vi "Autonomous Independent.vi"   [LabVIEW 2020]
doc: "This VI is called when autonomous begins, and will automatically be terminated when autonomous ends. You can carry out timed or sensor driven robot movement independently without needing to return to the caller."
uses:
  <vilib>/Rock Robotics/WPI/Solenoid/WPI_SolenoidValue.ctl
  <vilib>/Rock Robotics/Network Tables/NT Read String.vi
  <vilib>/Rock Robotics/Network Tables/NT Write String.vi
  Robot Global Data.vi
  <vilib>/Rock Robotics/WPI/Solenoid/WPI_SolenoidSetEnum.vi
  <vilib>/Rock Robotics/Network Tables/NT Write Numeric Array.vi
panel:
  # "Be sure to right-click and choose Data Operations>>Make Current Value default if you want to save the array values with the VI"
types:
  T1 = typedef "WPI_JoystickDevRef.ctl" = cluster{"Device":T2}
  T2 = typedef "WPI_JoystickDeviceEnum.ctl" = enum16{"USB 0", "USB 1", "USB 2", "USB 3", "USB 4", "USB 5"}
  T3 = enum16{"No-op", "Auto_Balance", "Arm_Setpoint", "Gripper", "Turn_IMU", "Drive_Distance", "Drive_to_Roll", "Stow_Intake", "Drive_to_GO", "Drive_to_Grid"}
  T4 = enum16{"Manual", "High Cone", "High Cube", "Mid Cone", "Mid Cube", "Intake", "Cube Handoff", "Cone Handoff", "Stow"}
  T5 = typedef "WPI_SolenoidValue.ctl" = enum16{"Off", "On", "Forward", "Reverse"}
  T6 = typedef "WPI_SolenoidDevRef.ctl" = cluster{"DevStatus":errorcluster, "Pneumatics Control Module":u8, "Forward Solenoid Channel":T7, "Reverse Solenoid Channel":T7}
  T7 = typedef "WPI_SolenoidChannel.ctl" = enum8{"Solenoid 0", "Solenoid 1", "Solenoid 2", "Solenoid 3", "Solenoid 4", "Solenoid 5", "Solenoid 6", "Solenoid 7", "Solenoid 8", "Solenoid 9", "Solenoid 10", "Solenoid 11", "Solenoid 12", "Solenoid 13", "Solenoid 14", "Solenoid 15", "Invalid"}
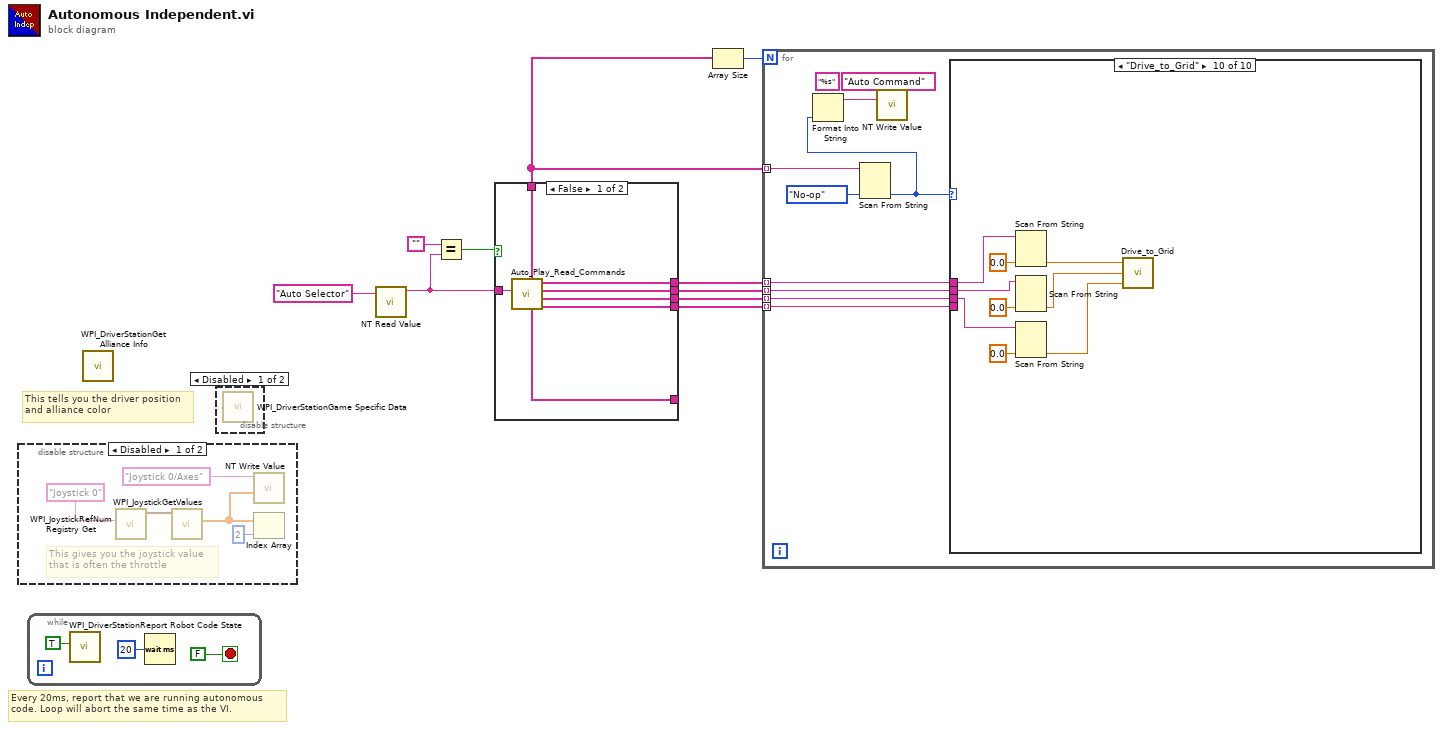
[diagram p0: block diagram]
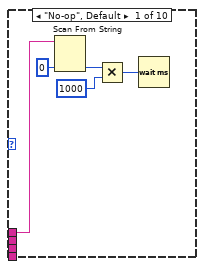
[diagram p2: hidden frame]
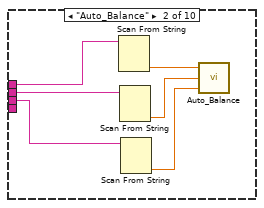
[diagram p3: hidden frame]
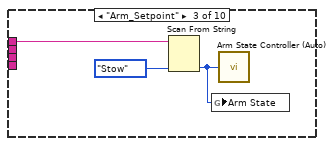
[diagram p4: hidden frame]
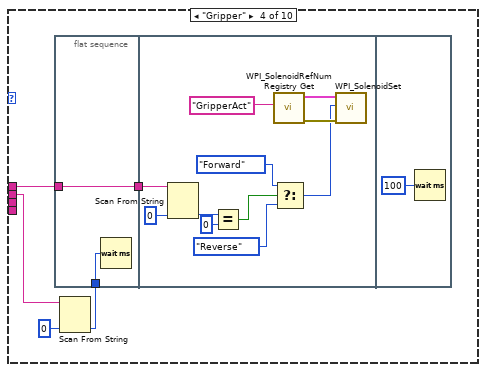
[diagram p5: hidden frame]
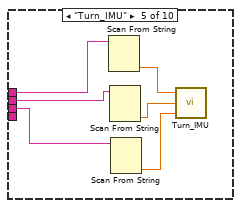
[diagram p6: hidden frame]
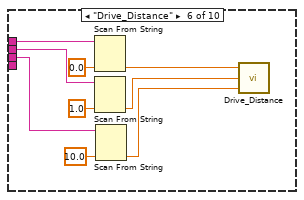
[diagram p7: hidden frame]
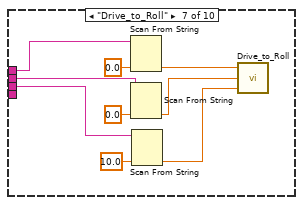
[diagram p8: hidden frame]
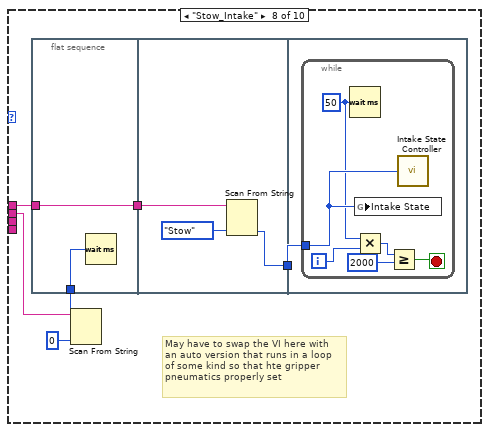
[diagram p9: hidden frame]
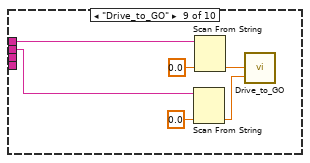
[diagram p10: hidden frame]
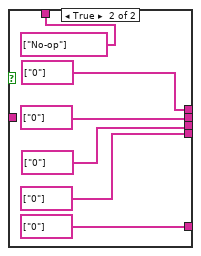
[diagram p11: hidden frame]
diagram:
  # "Every 20ms, report that we are running autonomous\ncode. Loop will abort the same time as the VI."
  # "This tells you the driver position\nand alliance color"
  n1 = disable-structure shown="Disabled" {
    frame Disabled {
      # "This gives you the joystick value\nthat is often the throttle"
      n2 = call <vilib>:"WPI_JoystickRefNum Registry Get.vi"("refnum name"="Joystick 0") -> ("JoystickDevRef"=w14:T1)  [unwired: 1 in, 9 out]
      n3 = call <vilib>:"WPI_JoystickGetValues.vi"("JoystickDevRef"=w14) -> ("Axes"=w12:dbl[])  [unwired: 6 in, 4 out]
      n4 = call-poly <vilib>:"NT Write Value.vi"("value"=w12, "name"="Joystick 0/Axes" ("Name")) -> ()  [unwired: 9 in, 1 out]
      n5 = Index Array(array=w12, index=2) -> ()  [unwired: 1 out]
    }
    frame Enabled {
    }
  }
  n6 = while {
    stop <- FALSE stop-if-true
    n7 = call <vilib>:"WPI_DriverStationReport Robot Code State.vi"("Autonomous"=TRUE) -> ()  [unwired: 10 in, 1 out]
    n8 = Wait (ms)(milliseconds to wait=u32 20) -> ()  [unwired: 1 out]
  }
  n9 = call <vilib>:"WPI_DriverStationGet Alliance Info.vi"() -> ()  [unwired: 12 out]
  n10 = disable-structure shown="Disabled" {
    frame Disabled {
      n11 = call <vilib>:"WPI_DriverStationGame Specific Data.vi"() -> ()  [unwired: 11 in, 1 out]
    }
    frame Enabled {
    }
  }
  n12 = call-poly <vilib>:"NT Read Value.vi"("name"="Auto Selector" ("Name")) -> ("value"=w7:string)  [unwired: 8 in, 2 out]
  n13 = Equal?(x="", y=w7) -> (x = y?=w8:bool)
  n14 = case shown="False" w8 {
    tunnel: w7 -> [w25 _]
    tunnel: [w24 string[] ["No-op"] ("Command Names")] -> w1
    tunnel: [w23 string[] ["0"] ("Parameter 1")] -> w5
    tunnel: [w22 string[] ["0"] ("Parameter 2")] -> w4
    tunnel: [w21 string[] ["0"] ("Parameter 3")] -> w3
    tunnel: [w20 string[] ["0"] ("Parameter 4")] -> w2
    tunnel: [w19 string[] ["0"] ("Concurrent?")] -> _
    frame False {
      n15 = call "Auto_Play_Read_Commands.vi"("Play Name"=w25) -> ("Parameter 4"=w20:string[], "Parameter 3"=w21:string[], "Parameter 2"=w22:string[], "Parameter 1"=w23:string[], "Concurrent?"=w19:string[], "Command Names"=w24:string[])  [unwired: 5 in]
    }
    frame True {
    }
  }
  n16 = Array Size(array=w1) -> (size(s)=w6:i32)
  n17 = for {
    N: w6 -> [_]
    tunnel: w5 -> [w38] mode=indexing
    tunnel: w4 -> [w37] mode=indexing
    tunnel: w3 -> [w36] mode=indexing
    tunnel: w2 -> [w35] mode=indexing
    tunnel: w1 -> [w40] mode=indexing
    (unwired) "%s" ("format string")
    n18 = Scan From String(input string=w40, default 1=T3."No-op") -> (output 1=w32:T3)  [unwired: 3 in, 3 out]
    n19 = Format Into String(w32) -> (resulting string=w33:string)  [unwired: 3 in, 1 out]
    n20 = call-poly <vilib>:"NT Write Value.vi"("value"=w33, "name"="Auto Command") -> ()  [unwired: 9 in, 1 out]
    n21 = case shown="\"Drive_to_Grid\"" w32 {
      tunnel: w38 -> [w45 w51 w54 w59 w79 w88 w97 w103 w121 w130]
      tunnel: w37 -> [_ w49 _ w57 w77 w86 w95 w101 w116 w128]
      tunnel: w36 -> [_ w47 _ _ w75 w82 w92 _ _ w125]
      tunnel: w35 -> [_ _ _ _ _ _ _ _ _ _]
      frame "No-op", Default {
        n22 = Scan From String(input string=w45, default 1=0) -> (output 1=w43:i32)  [unwired: 3 in, 3 out]
        n23 = Multiply(x=w43, y=1000) -> (x*y=w41:i32)
        n24 = Wait (ms)(milliseconds to wait=w41) -> ()  [unwired: 1 out]
      }
      frame "Auto_Balance" {
        n25 = Scan From String(input string=w51) -> (output 1=w50:dbl)  [unwired: 4 in, 3 out]
        n26 = Scan From String(input string=w49) -> (output 1=w48:dbl)  [unwired: 4 in, 3 out]
        n27 = Scan From String(input string=w47) -> (output 1=w46:dbl)  [unwired: 4 in, 3 out]
        n28 = call "Auto_Balance.vi"("Timeout (ms)"=w46, "Balance Complete Limit"=w48, "Kp"=w50) -> ()  [unwired: 1 in]
      }
      frame "Arm_Setpoint" {
        n29 = Scan From String(input string=w54, default 1=T4."Stow" ("Target Arm State")) -> (output 1=w52:T4)  [unwired: 3 in, 3 out]
        n30 = global write "Robot Global Data.vi" "Arm State"(w52) -> ()
        n31 = call "Arm State Controller (Auto).vi"("Target Arm State"=w52) -> ()
      }
      frame "Gripper" {
        n32 = flat-sequence {
          tunnel: w59 -> [w61]
          tunnel: [w61] -> w58
          tunnel: w55 -> [w60]
          tunnel: w58 -> [w71]
          frame #0 {
            n33 = Wait (ms)(milliseconds to wait=w60) -> ()  [unwired: 1 out]
          }
          frame #1 {
            n34 = Scan From String(input string=w71, default 1=0) -> (output 1=w69:i32)  [unwired: 3 in, 3 out]
            n35 = Equal?(x=w69, y=0) -> (x = y?=w67:bool)
            n36 = call <vilib>:"WPI_SolenoidRefNum Registry Get.vi"("refnum name"="GripperAct") -> ("error out"=w63:errorcluster, "SolenoidDevRef"=w64:T6)  [unwired: 9 in]
            n37 = Select(t=WPI_SolenoidValue."Forward" ("Value"), s=w67, f=WPI_SolenoidValue."Reverse" ("Value")) -> (s? t:f=w62:T5)
            n38 = call-poly <vilib>:"WPI_SolenoidSet.vi"("error in (no error)"=w63, "Value"=w62, "SolenoidDevRef"=w64) -> ()  [unwired: 7 in, 2 out]
          }
          frame #2 {
            n39 = Wait (ms)(milliseconds to wait=u32 100) -> ()  [unwired: 1 out]
          }
        }
        n40 = Scan From String(input string=w57, default 1=0) -> (output 1=w55:i32)  [unwired: 3 in, 3 out]
      }
      frame "Turn_IMU" {
        n41 = Scan From String(input string=w79) -> (output 1=w78:dbl)  [unwired: 4 in, 3 out]
        n42 = Scan From String(input string=w77) -> (output 1=w76:dbl)  [unwired: 4 in, 3 out]
        n43 = Scan From String(input string=w75) -> (output 1=w74:dbl)  [unwired: 4 in, 3 out]
        n44 = call "Turn_IMU.vi"("Timeout (s)"=w74, "Acceptable Error (Degrees)"=w76, "Target (Degrees)"=w78) -> ()
      }
      frame "Drive_Distance" {
        n45 = Scan From String(input string=w88, default 1=0.0 ("default value 1")) -> (output 1=w87:dbl)  [unwired: 3 in, 3 out]
        n46 = Scan From String(input string=w86, default 1=1.0 ("default value 1")) -> (output 1=w83:dbl)  [unwired: 3 in, 3 out]
        n47 = Scan From String(input string=w82, default 1=10.0 ("default value 1")) -> (output 1=w81:dbl)  [unwired: 3 in, 3 out]
        n48 = call "Drive_Distance.vi"("Timeout (ms)"=w81, "Acceptable Error (in)"=w83, "Distance (in)"=w87) -> ()  [unwired: 1 out]
      }
      frame "Drive_to_Roll" {
        n49 = Scan From String(input string=w97, default 1=0.0 ("default value 1")) -> (output 1=w96:dbl)  [unwired: 3 in, 3 out]
        n50 = Scan From String(input string=w95, default 1=0.0 ("default value 1")) -> (output 1=w94:dbl)  [unwired: 3 in, 3 out]
        n51 = Scan From String(input string=w92, default 1=10.0 ("default value 1")) -> (output 1=w93:dbl)  [unwired: 3 in, 3 out]
        n52 = call "Drive_to_Roll.vi"("Timeout (ms)"=w93, "Roll Cutoff (degrees)"=w94, "Distance Timeout (in)"=w96) -> ()  [unwired: 1 in]
      }
      frame "Stow_Intake" {
        # "May have to swap the VI here with\nan auto version that runs in a loop\nof some kind so that hte gripper\npneumatics properly set"
        n53 = flat-sequence {
          tunnel: w103 -> [w105]
          tunnel: [w105] -> w102
          tunnel: w99 -> [w104]
          tunnel: w102 -> [w108]
          tunnel: [w106] -> w98
          tunnel: w98 -> [w109]
          frame #0 {
            n54 = Wait (ms)(milliseconds to wait=w104) -> ()  [unwired: 1 out]
          }
          frame #1 {
            n55 = Scan From String(input string=w108, default 1=enum16{"Cone", "Cube", "Cube Handoff", "Stow"}."Stow" ("Intake State")) -> (output 1=w106:enum16{"Cone", "Cube", "Cube Handoff", "Stow"})  [unwired: 3 in, 3 out]
          }
          frame #2 {
            n56 = while {
              tunnel: w109 -> [w115]
              i -> [w112]
              stop <- w114 stop-if-true
              w111 = u32 50 ("milliseconds to wait")
              n57 = Wait (ms)(milliseconds to wait=w111) -> ()  [unwired: 1 out]
              n58 = global write "Robot Global Data.vi" "Intake State"(w115) -> ()
              n59 = Multiply(x=w111, y=w112) -> (x*y=w113:u32)
              n60 = Greater Or Equal?(x=w113, y=u32 2000) -> (x >= y?=w114:bool)
              n61 = call "Intake State Controller.vi"("Intake State"=w115) -> ()
            }
          }
        }
        n62 = Scan From String(input string=w101, default 1=0) -> (output 1=w99:i32)  [unwired: 3 in, 3 out]
      }
      frame "Drive_to_GO" {
        n63 = Scan From String(input string=w116, default 1=0.0 ("default value 1")) -> (output 1=w117:dbl)  [unwired: 3 in, 3 out]
        n64 = Scan From String(input string=w121, default 1=0.0 ("default value 1")) -> (output 1=w120:dbl)  [unwired: 3 in, 3 out]
        n65 = call "Drive_to_GO.vi"("Timeout (ms)"=w117, "Distance Timeout (in)"=w120) -> ()  [unwired: 1 in]
      }
      frame "Drive_to_Grid" {
        n66 = Scan From String(input string=w130, default 1=0.0 ("default value 1")) -> (output 1=w129:dbl)  [unwired: 3 in, 3 out]
        n67 = Scan From String(input string=w128, default 1=0.0 ("default value 1")) -> (output 1=w127:dbl)  [unwired: 3 in, 3 out]
        n68 = Scan From String(input string=w125, default 1=0.0 ("default value 1")) -> (output 1=w126:dbl)  [unwired: 3 in, 3 out]
        n69 = call "Drive_to_Grid.vi"("Timeout (ms)"=w126, "Distance from Target (m)"=w127, "Speed (m/s)"=w129) -> ()  [unwired: 1 in]
      }
    }
  }
